vi "_Convert Single Frame (Raw to CAN).vi"(7 "error in":errorcluster, 10 "Raw U32":u32[](array[numeric])=[0, 0, 66, 8, 167772160, 0] format="%.0x") -> (0 "error out":errorcluster, 3 "CAN frame":T1 {"payload" format="%x"; "timestamp" format="%<%.7X\n%x>T"; "type" items=["CAN Data"=0, "CAN Remote"=1, "CAN Bus Error"=2, "CAN 2.0 Data"=8, "CAN FD Data"=16, "CAN FD+BRS Data"=24, "J1939 Data"=192, "Delay"=224, "Log Trigger"=225, "Start Trigger"=226]; "identifier" format="%x"})   [LabVIEW 2020, in "985x Support Addon Engine.lvlib"]
doc: "Convert array of raw frame data to a single CAN frame.\n\nIf no valid frame exists at the current index, the boolean \"valid?\" is false.\n\nUpon return, index is set to the start of the next CAN frame in raw data, or -1 if the end of the raw data was reached."
uses:
  985x Support Addon Engine.lvlib
  <vilib>/xnet/xnet.llb/XNET Frame Type CAN.ctl
  <vilib>/xnet/xnet.llb/XNET Frame CAN.ctl
panel:
  # "Timestamp conversion might be incorrect."
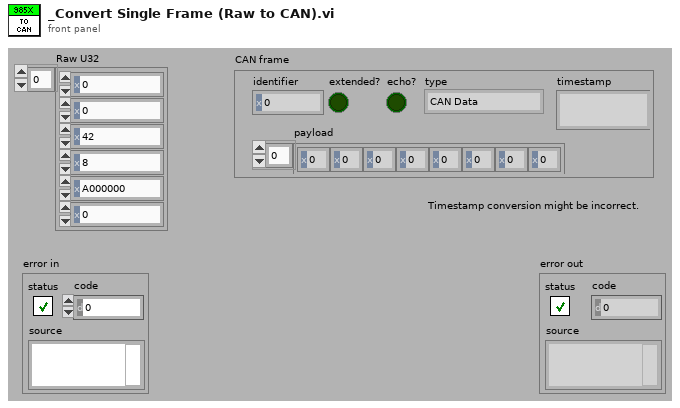
[diagram p1: front panel]
types:
  T1 = typedef "XNET Frame CAN.ctl" = cluster{"timestamp":timestamp, "payload":u8[], "identifier":u32, "type":T2, "extended?":bool, "echo?":bool}
  T2 = typedef "XNET Frame Type CAN.ctl" = u8
  T3 = enum16{"big-endian, network order", "native, host order", "little-endian"}
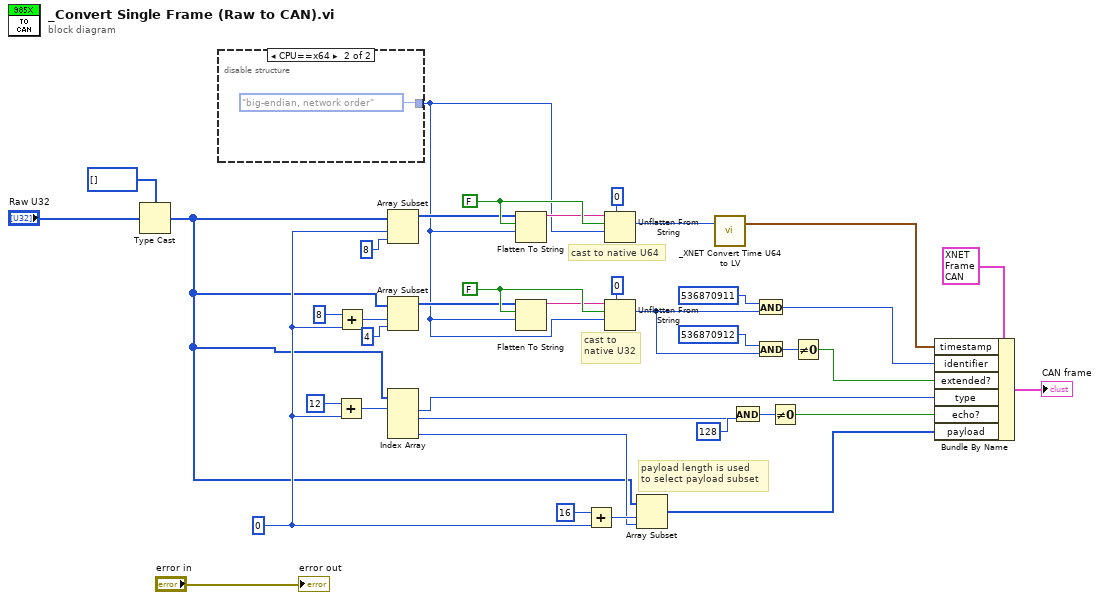
[diagram p0: block diagram]
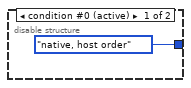
[diagram p2: hidden frame]
diagram:
  w7 = 0
  w17 = FALSE ("prepend array or string size? (T)")
  w22 = FALSE ("prepend array or string size? (T)")
  # "payload length is used\nto select payload subset"
  # "cast to \nnative U32"
  # "cast to native U64"
  n1 = Type Cast(type=u8[] [] ("raw frames"), x="Raw U32") -> (*(type *) &x=w2:u8[])
  n2 = disable-structure shown="CPU==x64" {
    disable-tunnel: [T3."native, host order" ("byte order (0:big-endian, network order)") T3."big-endian, network order" ("byte order (0:big-endian, network order)")] -> w4
    frame condition #0 (active) {
    }
    frame condition #1 {
    }
  }
  n3 = Add(x=12, y=w7) -> (x+y=w27:i32)
  n4 = Add(x=8, y=w7) -> (x+y=w29:i32)
  n5 = Array Subset(array=w2, index=w7, length=8) -> (w15:u8[])
  n6 = Array Subset(array=w2, index=w29, length=4) -> (w20:u8[])
  n7 = Index Array(array=w2, index #1=w27) -> (element #1=w26:u8, element #2=w9:u8, element #4=w23:u8)  [unwired: 3 in, 1 out]
  n8 = Flatten To String(anything=w15, prepend array or string size? (T)=w17, byte order (0:big-endian, network order)=w4) -> (data string=w16:string)  [unwired: 1 in, 2 out]
  n9 = Flatten To String(anything=w20, prepend array or string size? (T)=w22, byte order (0:big-endian, network order)=w4) -> (data string=w21:string)  [unwired: 1 in, 2 out]
  n10 = Add(x=16, y=w7) -> (x+y=w24:i32)
  n11 = Unflatten From String(type=u64 0 ("length"), binary string=w16, data includes array or string size? (T)=w17, byte order (0:big-endian, network order)=w4) -> (value=w13:u64)  [unwired: 1 in, 2 out]
  n12 = Unflatten From String(type=u32 0 ("length"), binary string=w21, data includes array or string size? (T)=w22, byte order (0:big-endian, network order)=w4) -> (value=w18:u32)  [unwired: 1 in, 2 out]
  n13 = Array Subset(array=w2, index=w24, length=w23) -> (w12:u8[])
  n14 = call <vilib>:"_XNET Convert Time U64 to LV.vi"("Time U64"=w13) -> ("Time LV"=w38:timestamp)  [unwired: 2 out]
  n15 = And(x=w9, y=u8 128) -> (x .and. y?=w11:u8)
  n16 = And(x=u32 536870911, y=w18) -> (x .and. y?=w35:u32)
  n17 = And(x=u32 536870912, y=w18) -> (x .and. y?=w34:u32)
  n18 = Not Equal To 0?(x=w11) -> (x != 0?=w8:bool)
  n19 = Not Equal To 0?(x=w34) -> (x != 0?=w33:bool)
  n20 = Bundle By Name(cluster=T1 {"timestamp"=timestamp(0 s since 1904-01-01), "payload"=[0, 0, 0, 0, 0, 0, 0, 0], "identifier"=0, "type"=0, "extended?"=FALSE, "echo?"=FALSE} ("CAN frame"), "timestamp"=w38, "identifier"=w35, "extended?"=w33, "type"=w26, "echo?"=w8, "payload"=w12) -> (→"CAN frame":T1)
  "error out" <- "error in"
